vi "To and From Array Test.vi"() -> (0 "error out":errorcluster, 2 "Lines Equal":bool, 3 "Class Equal":bool)   [LabVIEW 2014, in "UI Reference tests.lvlib"]
uses:
  UI Reference tests.lvlib
  module/configuration/UI Reference configuration.lvclass/UI Reference configuration.ctl
  <vilib>/NI/Tag Bus Module Framework/channel/TBM channel.lvclass
  module/configuration/UI Reference configuration.lvclass
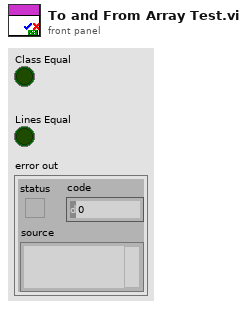
[diagram p1: front panel]
types:
  T1 = typedef "UI Reference configuration.lvclass/Line.ctl" = cluster{"channel":refnum<class "TBM channel.lvclass">}
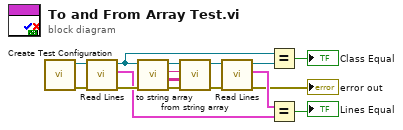
[diagram p0: block diagram]
diagram:
  n1 = call "Create Test Configuration.vi"() -> ("error out"=w8:errorcluster, "Module Configuration"=w9:refnum<class "UI Reference configuration.lvclass">)  [unwired: 6 in, 4 out]
  n2 = call "Read Lines.vi"("error in (no error)"=w8, "UI Reference configuration in"=w9) -> ("error out"=w10:errorcluster, "Lines"=w4:T1[], "UI Reference configuration out"=w6:refnum<class "UI Reference configuration.lvclass">)  [unwired: 7 in]
  n3 = call-dynamic "to string array.vi"("error in (no error)"=w10, "UI Reference configuration in"=w6) -> ("error out"=w16:errorcluster, "Array"=w15:string[][], "version"=w14:string, "UI Reference configuration out"=w13:refnum<class "UI Reference configuration.lvclass">)  [unwired: 6 in]
  n4 = call-dynamic "from string array.vi"("error in (no error)"=w16, "String Array"=w15, "version"=w14, "UI Reference configuration in"=w13) -> ("error out"=w11:errorcluster, "UI Reference configuration out"=w12:refnum<class "UI Reference configuration.lvclass">)  [unwired: 6 in]
  n5 = call "Read Lines.vi"("error in (no error)"=w11, "UI Reference configuration in"=w12) -> ("error out"=→"error out":errorcluster, "Lines"=w5:T1[], "UI Reference configuration out"=w7:refnum<class "UI Reference configuration.lvclass">)  [unwired: 7 in]
  n6 = Equal?(x=w6, y=w7) -> (x = y?=→"Class Equal":bool)
  n7 = Equal?(x=w5, y=w4) -> (x = y?=→"Lines Equal":bool)
